vi "tuneLeftOpenLoop_DriveQuadTalonSRX.vi"(11 "F Open Loop R":dbl=0.92 format="%.5f") -> ()   [LabVIEW 2019, in "DriveQuadTalonSRX_Motor.lvlib"]
uses:
  DriveQuadTalonSRX_Motor.lvlib
  globals_DriveQuadTalonSRX.vi
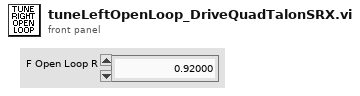
[diagram p1: front panel]
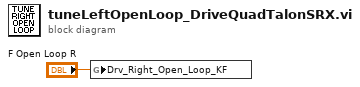
[diagram p0: block diagram]
diagram:
  n1 = global write "globals_DriveQuadTalonSRX.vi" "Drv_Right_Open_Loop_KF"("F Open Loop R") -> ()
